vi "Inverter Adjust.vi"(8 "error in":errorcluster, 11 "DAC Inverter in":refnum<class "DAC Inverter.lvclass">) -> (0 "error out":errorcluster, 3 "DAC Inverter out":refnum<class "DAC Inverter.lvclass">)   [LabVIEW 2019, in "DAC.lvlib" / "DAC Inverter.lvclass"]
uses:
  DAC Inverter.lvclass
  Results/Results Method.ctl
  Results/DeepU Results/DeepU Results.lvclass
  DAC Inverter.lvclass/DAC Inverter.ctl
  Results/DeepU Results/DeepU Results.lvclass/DeepU Results.ctl
  <vilib>/NI/Modbus Library/API/Master/Modbus Master.lvclass
  Results/Results.lvlib
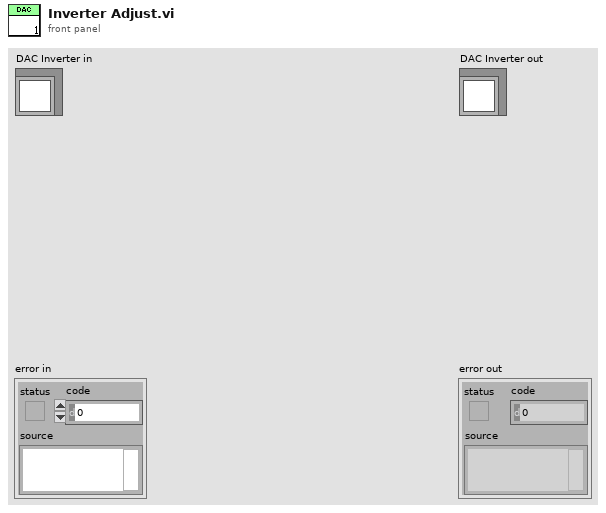
[diagram p1: front panel]
types:
  T1 = typedef "Results.lvlib/Results Method.ctl" = enum16{"Get", "Set"}
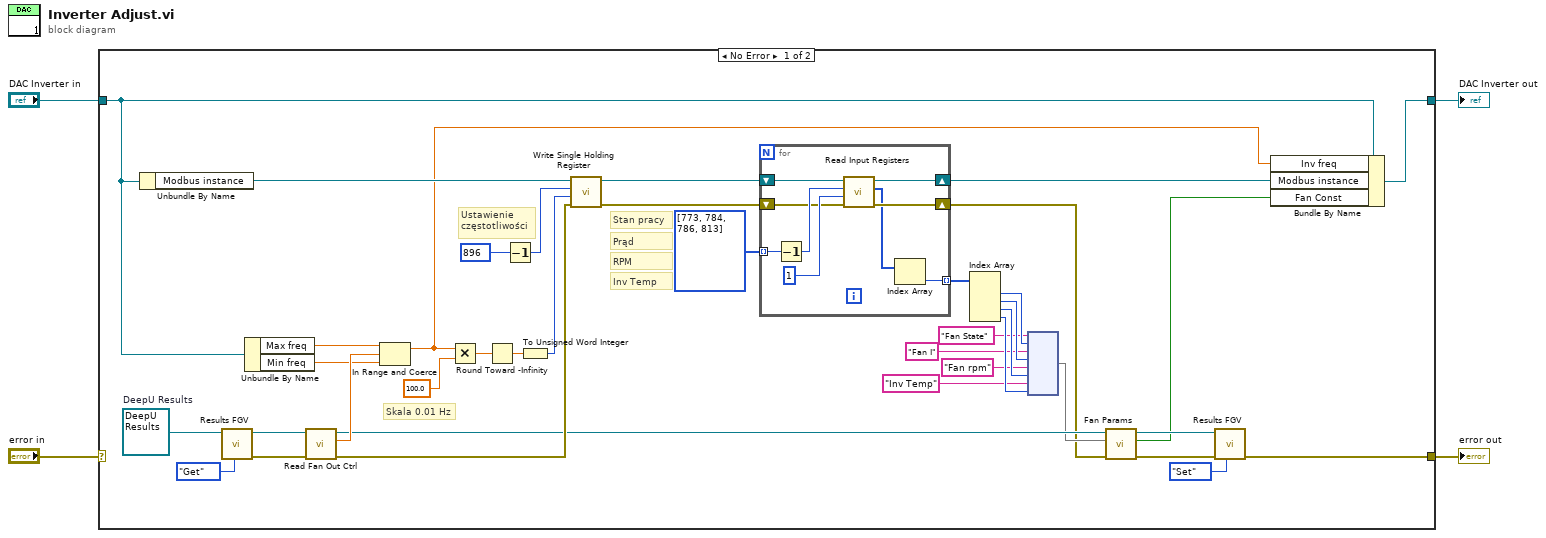
[diagram p0: block diagram]
diagram:
  n1 = case shown="No Error" "error in" {
    selector: "error in" -> [_ w54]
    tunnel: [w25 w54] -> w3
    tunnel: [w37 w53] -> w1
    tunnel: "DAC Inverter in" -> [w32 w53]
    frame No Error {
      w43 = refnum<class "DeepU Results.lvclass"> refnum  # DeepU Results
      # "Inv Temp"
      # "RPM"
      # "Prąd"
      # "Stan pracy"
      # "Skala 0.01 Hz"
      # "Ustawienie\nczęstotliwości"
      n2 = Unbundle By Name(w32) -> ("Modbus instance"=w38:refnum<class "Modbus Master.lvclass">)
      n3 = call-dynamic "Results FGV.vi"("Method"=Results_Method."Get", "DeepU Results in"=w43) -> ("error out"=w35:errorcluster, "DeepU Results out"=w36:refnum<class "DeepU Results.lvclass">)  [unwired: 8 in]
      n4 = Unbundle By Name(w32) -> ("Max freq"=w31:dbl, "Min freq"=w30:dbl)
      n5 = call "Read Fan Out Ctrl.vi"("error in (no error)"=w35, "DeepU Results in"=w36) -> ("error out"=w26:errorcluster, "Fan Out Ctrl"=w33:dbl, "DeepU Results out"=w21:refnum<class "DeepU Results.lvclass">)  [unwired: 7 in]
      n6 = In Range and Coerce(upper limit=w31, x=w33, lower limit=w30) -> (coerced(x)=w17:dbl)  [unwired: 1 out]
      n7 = Multiply(x=w17, y=100.0) -> (x*y=w29:dbl)
      n8 = Round Toward -Infinity(1:w29) -> (0:w28:dbl)
      n9 = Decrement(x=u16 896 ("address")) -> (x-1=w39:u16)
      n10 = To Unsigned Word Integer(number=w28) -> (unsigned 16bit integer=w27:u16)
      n11 = call-dynamic "Write Single Holding Register.vi"("error in"=w26, "register to write"=w27, "address"=w39, "Modbus master in"=w38) -> ("error out"=w23:errorcluster, "Modbus master out"=w24:refnum<class "Modbus Master.lvclass">)  [unwired: 6 in]
      n12 = for {
        tunnel: u16[] [773, 784, 786, 813] -> [w50] mode=indexing
        shift-right: [w47] -> w22
        shift-left: w24 -> [w51]
        shift-right: [w46] -> w6
        shift-left: w23 -> [w48]
        tunnel: [w44] -> w16 mode=indexing
        n13 = Decrement(x=w50) -> (x-1=w52:u16)
        n14 = call-dynamic "Read Input Registers.vi"("error in"=w48, "number of inputs"=u16 1, "starting address"=w52, "Modbus master in"=w51) -> ("error out"=w46:errorcluster, "register values"=w45:u16[], "Modbus master out"=w47:refnum<class "Modbus Master.lvclass">)  [unwired: 5 in]
        n15 = Index Array(array=w45) -> (element=w44:u16)  [unwired: 1 in]
      }
      n16 = Index Array(array=w16) -> (element #1=w15:u16, element #2=w14:u16, element #3=w13:u16, element #4=w12:u16)  [unwired: 4 in]
      n17 = node("Fan State" ("key"), w15, "Fan I" ("key"), w14, "Fan rpm" ("key"), w13, "Inv Temp" ("key"), w12) -> (w7:map{string, u16})
      n18 = call "Fan Params.vi"("error in"=w6, "Fan Params Registers"=w7, "DeepU Results in"=w21) -> ("error out"=w19:errorcluster, "Fan Const"=w5:bool, "DeepU Results out"=w20:refnum<class "DeepU Results.lvclass">)  [unwired: 6 in]
      n19 = call-dynamic "Results FGV.vi"("Method"=Results_Method."Set", "error in"=w19, "DeepU Results in"=w20) -> ("error out"=w25:errorcluster)  [unwired: 7 in, 1 out]
      n20 = Bundle By Name(cluster=w32, "Inv freq"=w17, "Modbus instance"=w22, "Fan Const"=w5) -> (w37:refnum<class "DAC Inverter.lvclass">)
    }
    frame Error {
    }
  }
  "error out" <- w3
  "DAC Inverter out" <- w1
